vi "DriveBaseTankDrive.vi"() -> ()   [LabVIEW 2016, in "DriveBase.lvclass"]
uses:
  DriveBase.lvclass
panel:
  out "DriveBase.lvclass 2":refnum<class "DriveBase.lvclass">
  in  "Y Axis":dbl
  in  "X Axis":dbl
  in  "DriveBase.lvclass":refnum<class "DriveBase.lvclass">
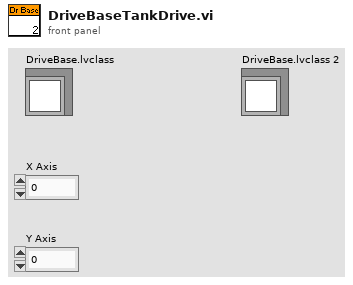
[diagram p1: front panel]
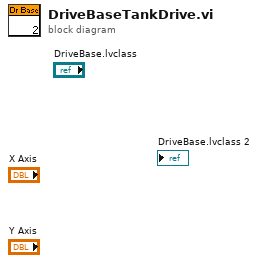
[diagram p0: block diagram]
diagram:
